vi "Check Redraw.vi"(8 "error in (no error)":errorcluster, 11 "HistorianCharting in":refnum<class "HistorianCharting.lvclass">) -> (0 "error out":errorcluster, 3 "HistorianCharting out":refnum<class "HistorianCharting.lvclass">)   [LabVIEW 2020, in "VolatusGUIElements.lvlib" / "HistorianCharting.lvclass"]
uses:
  HistorianCharting.lvclass
  HistorianCharting.lvclass/HistorianCharting.ctl
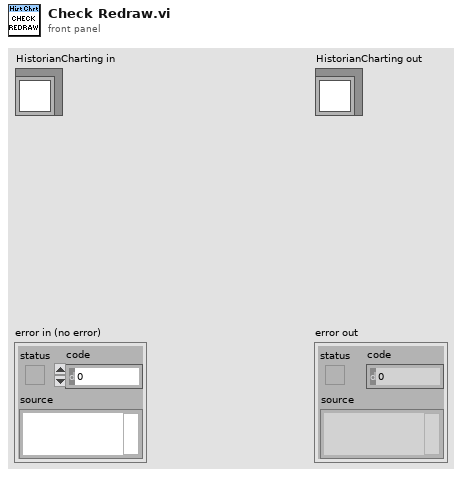
[diagram p1: front panel]
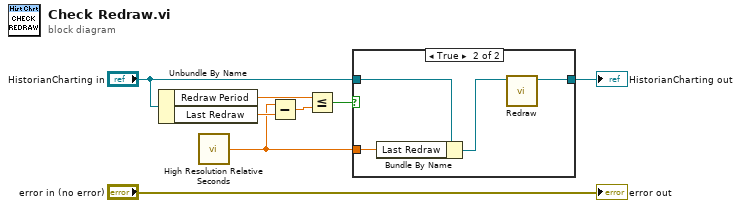
[diagram p0: block diagram]
diagram:
  n1 = Unbundle By Name("HistorianCharting in") -> ("Redraw Period"=w4:dbl, "Last Redraw"=w6:dbl)
  n2 = call <vilib>:"High Resolution Relative Seconds.vi"() -> ("relative seconds"=w1:dbl)
  n3 = Subtract(x=w1, y=w6) -> (x-y=w5:dbl)
  n4 = Less Or Equal?(x=w4, y=w5) -> (x <= y?=w2:bool)
  n5 = case shown="True" w2 {
    tunnel: "HistorianCharting in" -> [w9 w13]
    tunnel: [w9 w12] -> w3
    tunnel: w1 -> [_ w10]
    frame False {
    }
    frame True {
      n6 = Bundle By Name(cluster=w13, "Last Redraw"=w10) -> (w11:refnum<class "HistorianCharting.lvclass">)
      n7 = call "Redraw.vi"("HistorianCharting in"=w11) -> ("HistorianCharting out"=w12:refnum<class "HistorianCharting.lvclass">)  [unwired: 9 in, 1 out]
    }
  }
  "HistorianCharting out" <- w3
  "error out" <- "error in (no error)"
